vi "CD Init_Prepare Async Data.vi"(8 "error in (no error)":errorcluster, 10 "Card Parameters (in)":T1, 11 "Channels In":T15[](array[typedef]) {"RTs"."Mode Codes"."Words Item Refs" format="%.0x"; "RTs"."Mode Codes"."Timestamp Channel Data Reference" format="%.0x"; "RTs"."subAddresses"."Words Item Refs" format="%.0x"; "RTs"."subAddresses"."Timestamp Channel Data Reference" format="%.0x"; "RTs"."Status Channel Data Reference" format="%.0x"; "RTs"."Command Channels Refs" format="%.0x"; "BC"."Acyclic Frames Trigger Channels Refs" format="%.0x"; "BC"."Command Channels Refs" format="%.0x"; "BC"."messages"."Timestamp Channel Data Reference" format="%.0x"; "BC"."messages"."Status Channel Data Refs" format="%.0x"; "BC"."messages"."Words Item Refs" format="%.0x"; "BC"."messages"."Words Block Data Refs"."Data Reference" format="%.0x"}) -> (0 "error out":errorcluster, 3 "RT Async Data":T3 {"Map (MC Tx)"."Word Data Reference" format="%.0x"; "Map (MC Rx)"."Channel Data Reference" format="%.0x"; "Map (RT Command Channels)"."RT Command Channel Ref" format="%.0x"; "MAP (BC Acyclic Messages Trigger)"."Acyclic Message Trigger Channel Ref" format="%.0x"; "Map (Bc Command Channels)"."BC Command Channel Ref" format="%.0x"; "Map (RT to ..)"."Word Data Reference" format="%.0x"; "Map (BC to RT)"."Channel Data Reference" format="%.0x"})   [LabVIEW 2017, in "Ballard MIL-1553 Engine.lvlib"]
uses:
  Ballard MIL-1553 Engine.lvlib
  Shared/Controls and Global/RT Channel.ctl
  Shared/Controls and Global/RT BC.ctl
  <vilib>/NI Veristand/Custom Device API/Custom Device Item Ref.ctl
  Shared/Controls and Global/RT Message.ctl
  Shared/Controls and Global/RT messageType.ctl
  Shared/Controls and Global/RT CWD1.ctl
  Shared/Controls and Global/RT CWD2.ctl
  <vilib>/NI Veristand/Custom Device API/Data Reference.ctl
  <vilib>/NI Veristand/Custom Device API/Block Data Reference.ctl
  Shared/Controls and Global/RT Remote Terminal.ctl
  Shared/Controls and Global/RT Remote Terminal_rtMode.ctl
  Shared/Controls and Global/RT Remote Terminal_RT subAddress.ctl
  Shared/Controls and Global/RT Remote Terminal_RT direction.ctl
  Shared/Controls and Global/RT Remote Terminal_RT Mode Code.ctl
  Controls/RT Async Data.ctl
  Controls/RT Async_Map BC2RT.ctl
  Controls/RT Async_Map_Type.ctl
  Controls/RT Async_Raw Values.ctl
  Controls/RT Async_Raw Values to Messages Index_Association.ctl
  Controls/RT Async_Map RT2BC.ctl
  Controls/RT Async_Map RTs Status.ctl
  Controls/RT Async_Map BC Command Channels.ctl
  Controls/RT Async_Map BC Acyclic Messages Trigger.ctl
  Controls/RT Async_Map RT Command Channels.ctl
  Controls/Card Parameters.ctl
  Shared/Controls and Global/Initialization Method.ctl
  <vilib>/NI VeriStand/Custom Device API/Custom Device API.lvlib
  Shared/Ballard 1553 Shared.lvlib
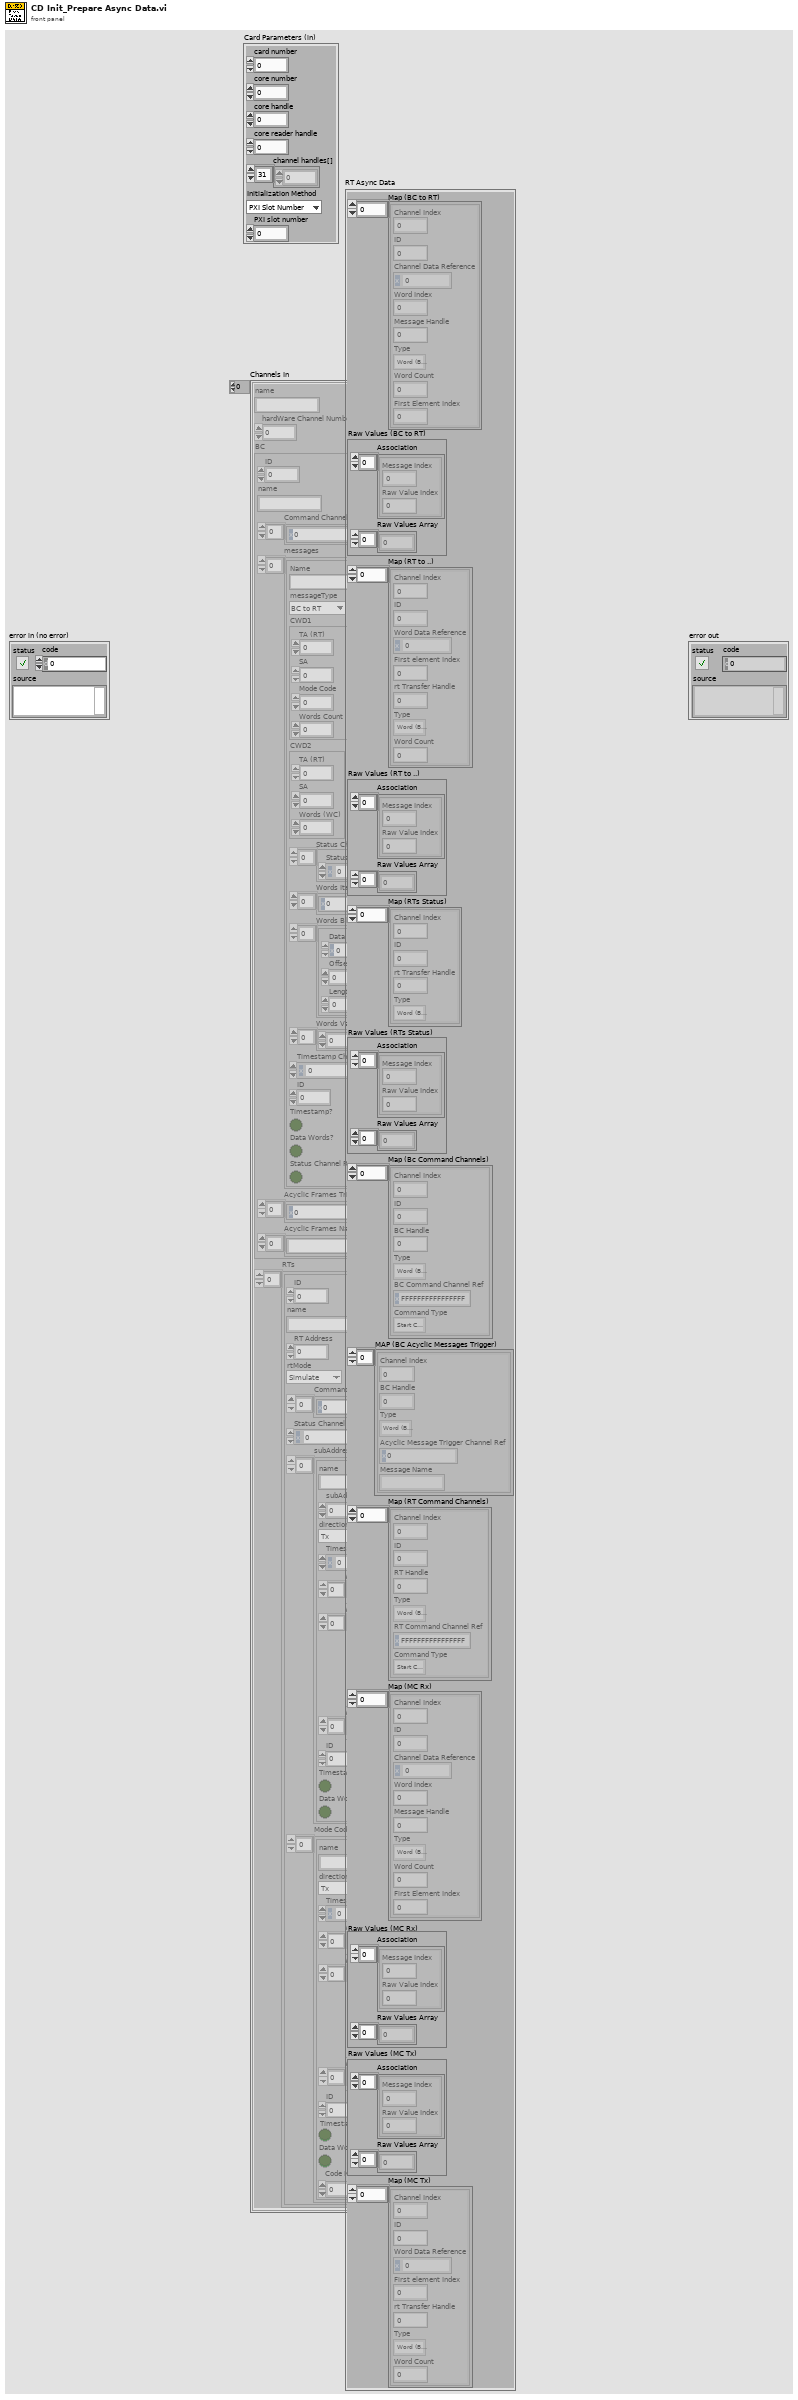
[diagram p1: front panel]
types:
  T1 = typedef "Ballard MIL-1553 Engine.lvlib/Card Parameters.ctl" = cluster{"card number":i32, "core number":i32, "core handle":u64, "core reader handle":u64, "channel handles[]":u64[], "Initialization Method":T2, "PXI slot number":i32}
  T2 = typedef "Ballard 1553 Shared.lvlib/Initialization Method.ctl" = enum16{"PXI Slot Number", "Card Number"}
  T3 = typedef "Ballard MIL-1553 Engine.lvlib/RT Async Data.ctl" = cluster{"Map (BC to RT)":T4[], "Raw Values (BC to RT)":T7, "Map (RT to ..)":T9[], "Raw Values (RT to ..)":T7, "Map (RTs Status)":T10[], "Raw Values (RTs Status)":T7, "Map (Bc Command Channels)":T11[], "MAP (BC Acyclic Messages Trigger)":T13[], "Map (RT Command Channels)":T14[], "Map (MC Rx)":T4[], "Raw Values (MC Rx)":T7, "Raw Values (MC Tx)":T7, "Map (MC Tx)":T9[]}
  T4 = typedef "Ballard MIL-1553 Engine.lvlib/RT Async_Map BC2RT.ctl" = cluster{"Channel Index":i32, "ID":i32, "Channel Data Reference":T5, "Word Index":i32, "Message Handle":u64, "Type":T6, "Word Count":i32, "First Element Index":i32}
  T5 = typedef "Custom Device API.lvlib/Data Reference.ctl" = i32
  T6 = typedef "Ballard MIL-1553 Engine.lvlib/RT Async_Map_Type.ctl" = enum16{"Word (BC to RT)", "Word (MC (Rx))", "Acyclic Message Trigger", "Word (RT to ..)", "Word (RT to RT)", "Word (MC (Tx))", "RT Status", "BC Commands", "RT Commands"}
  T7 = typedef "Ballard MIL-1553 Engine.lvlib/RT Async_Raw Values.ctl" = cluster{"Association":T8[], "Raw Values Array":u16[]}
  T8 = typedef "Ballard MIL-1553 Engine.lvlib/RT Async_Raw Values to Messages Index_Association.ctl" = cluster{"Message Index":i32, "Raw Value Index":i32}
  T9 = typedef "Ballard MIL-1553 Engine.lvlib/RT Async_Map RT2BC.ctl" = cluster{"Channel Index":i32, "ID":i32, "Word Data Reference":T5, "First element Index":i32, "rt Transfer Handle":u64, "Type":T6, "Word Count":i32}
  T10 = typedef "Ballard MIL-1553 Engine.lvlib/RT Async_Map RTs Status.ctl" = cluster{"Channel Index":i32, "ID":i32, "rt Transfer Handle":u64, "Type":T6}
  T11 = typedef "Ballard MIL-1553 Engine.lvlib/RT Async_Map BC Command Channels.ctl" = cluster{"Channel Index":i32, "ID":i32, "BC Handle":u64, "Type":T6, "BC Command Channel Ref":T12, "Command Type":enum16{"Start Command", "Stop Command"}}
  T12 = typedef "Custom Device API.lvlib/Custom Device Item Ref.ctl" = u64
  T13 = typedef "Ballard MIL-1553 Engine.lvlib/RT Async_Map BC Acyclic Messages Trigger.ctl" = cluster{"Channel Index":i32, "BC Handle":u64, "Type":T6, "Acyclic Message Trigger Channel Ref":T12, "Message Name":string}
  T14 = typedef "Ballard MIL-1553 Engine.lvlib/RT Async_Map RT Command Channels.ctl" = cluster{"Channel Index":i32, "ID":i32, "RT Handle":u64, "Type":T6, "RT Command Channel Ref":T12, "Command Type":enum16{"Start Command", "Stop Command"}}
  T15 = typedef "Ballard 1553 Shared.lvlib/RT Channel.ctl" = cluster{"name":string, "hardWare Channel Number":u16, "BC":T16, "RTs":T22[]}
  T16 = typedef "Ballard 1553 Shared.lvlib/RT BC.ctl" = cluster{"ID":i32, "name":string, "Command Channels Refs":T12[], "messages":T17[], "Acyclic Frames Trigger Channels Refs":T12[], "Acyclic Frames Names":string[]}
  T17 = typedef "Ballard 1553 Shared.lvlib/RT Message.ctl" = cluster{"Name":string, "messageType":T18, "CWD1":T19, "CWD2":T20, "Status Channel Data Refs":T5[], "Words Item Refs":T12[], "Words Block Data Refs":T21[], "Words Values Array":u16[], "Timestamp Channel Data Reference":T5, "ID":i32, "Timestamp?":bool, "Data Words?":bool, "Status Channel Ref?":bool}
  T18 = typedef "Ballard 1553 Shared.lvlib/RT messageType.ctl" = enum16{"BC to RT", "RT to BC", "RT to RT", "MC (Rx)", "MC (Tx)"}
  T19 = typedef "Ballard 1553 Shared.lvlib/RT CWD1.ctl" = cluster{"TA (RT)":i8, "SA":i8, "Mode Code":i8, "Words Count":i8}
  T20 = typedef "Ballard 1553 Shared.lvlib/RT CWD2.ctl" = cluster{"TA (RT)":i8, "SA":i8, "Words (WC)":i8}
  T21 = typedef "Custom Device API.lvlib/Block Data Reference.ctl" = cluster{"Data Reference":T5, "Offset":u64, "Length":u64}
  T22 = typedef "Ballard 1553 Shared.lvlib/RT Remote Terminal.ctl" = cluster{"ID":i32, "name":string, "RT Address":i32, "rtMode":T23, "Command Channels Refs":T12[], "Status Channel Data Reference":T5, "subAddresses":T24[], "Mode Codes":T26[]}
  T23 = typedef "Ballard 1553 Shared.lvlib/RT Remote Terminal_rtMode.ctl" = enum16{"Simulate", "Monitor", "Disable"}
  T24 = typedef "Ballard 1553 Shared.lvlib/RT Remote Terminal_RT subAddress.ctl" = cluster{"name":string, "subAddress":i8, "direction":T25, "Timestamp Channel Data Reference":T5, "Words Values Array":u16[], "Words Block Data Refs":T21[], "Words Item Refs":T12[], "ID":i32, "Timestamp?":bool, "Data Words?":bool}
  T25 = typedef "Ballard 1553 Shared.lvlib/RT Remote Terminal_RT direction.ctl" = enum16{"Tx", "Rx"}
  T26 = typedef "Ballard 1553 Shared.lvlib/RT Remote Terminal_RT Mode Code.ctl" = cluster{"name":string, "direction":T25, "Timestamp Channel Data Reference":T5, "Words Values Array":u16[], "Words Block Data Refs":T21[], "Words Item Refs":T12[], "ID":i32, "Timestamp?":bool, "Data Words?":bool, "Code Number":i32}
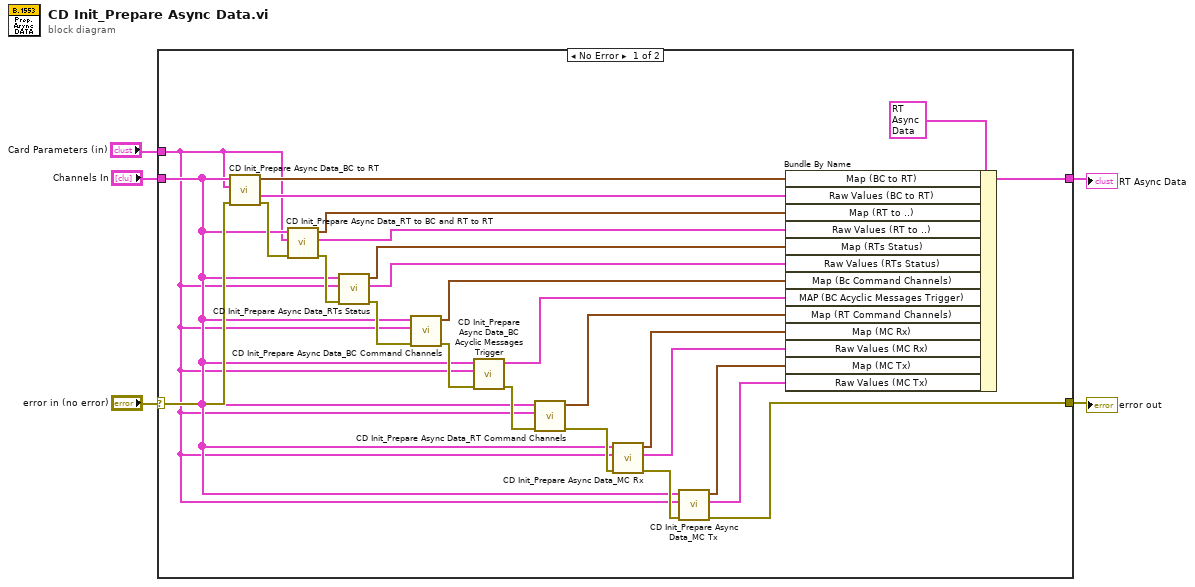
[diagram p0: block diagram]
diagram:
  n1 = case shown="No Error" "error in (no error)" {
    selector: "error in (no error)" -> [w30 w32]
    tunnel: [w10 w32] -> w4
    tunnel: "Channels In" -> [w7 _]
    tunnel: "Card Parameters (in)" -> [w6 _]
    tunnel: [w31 _] -> w1
    frame No Error {
      n2 = call "CD Init_Prepare Async Data_BC to RT.vi"("error in (no error)"=w30, "Card Parameters (in)"=w6, "Channels In"=w7) -> ("error out"=w24:errorcluster, "Raw Values (BC to RT)"=w27:T7, "Map (BC to RT)"=w28:T4[])  [unwired: 6 in]
      n3 = call "CD Init_Prepare Async Data_RT to BC and RT to RT.vi"("error in (no error)"=w24, "Card Parameters (in)"=w6, "Channels In"=w7) -> ("error out"=w23:errorcluster, "Raw Values (RT to BC)"=w25:T7, "Map (RT to BC)"=w26:T9[])  [unwired: 6 in]
      n4 = call "CD Init_Prepare Async Data_RTs Status.vi"("error in (no error)"=w23, "Card Parameters (in)"=w6, "Channels In"=w7) -> ("error out"=w20:errorcluster, "Raw Values (RTs Status)"=w21:T7, "Map (RTs Status)"=w22:T10[])  [unwired: 6 in]
      n5 = call "CD Init_Prepare Async Data_BC Command Channels.vi"("error in (no error)"=w20, "Card Parameters (in)"=w6, "Channels In"=w7) -> ("error out"=w18:errorcluster, "Map (Bc Command Channels)"=w19:T11[])  [unwired: 7 in]
      n6 = call "CD Init_Prepare Async Data_BC Acyclic Messages Trigger.vi"("error in (no error)"=w18, "Card Parameters (in)"=w6, "Channels In"=w7) -> ("error out"=w17:errorcluster, "MAP (BC Acyclic Messages Trigger)"=w16:T13[])  [unwired: 7 in]
      n7 = call "CD Init_Prepare Async Data_RT Command Channels.vi"("error in (no error)"=w17, "Card Parameters (in)"=w6, "Channels In"=w7) -> ("error out"=w14:errorcluster, "Map (RT Command Channels)"=w15:T14[])  [unwired: 7 in]
      n8 = call "CD Init_Prepare Async Data_MC Rx.vi"("error in (no error)"=w14, "Card Parameters (in)"=w6, "Channels In"=w7) -> ("error out"=w11:errorcluster, "Raw Values (MC Rx)"=w12:T7, "Map (MC Rx)"=w13:T4[])  [unwired: 6 in]
      n9 = call "CD Init_Prepare Async Data_MC Tx.vi"("error in (no error)"=w11, "Card Parameters (in)"=w6, "Channels In"=w7) -> ("error out"=w10:errorcluster, "Raw Values (RT to BC)"=w8:T7, "Map (MC Tx)"=w9:T9[])  [unwired: 6 in]
      n10 = Bundle By Name(cluster=T3 {"Map (BC to RT)"=[], "Raw Values (BC to RT)"={"Association"=[], "Raw Values Array"=[]}, "Map (RT to ..)"=[], "Raw Values (RT to ..)"={"Association"=[], "Raw Values Array"=[]}, "Map (RTs Status)"=[], "Raw Values (RTs Status)"={"Association"=[], "Raw Values Array"=[]}, "Map (Bc Command Channels)"=[], "MAP (BC Acyclic Messages Trigger)"=[], "Map (RT Command Channels)"=[], "Map (MC Rx)"=[], "Raw Values (MC Rx)"={"Association"=[], "Raw Values Array"=[]}, "Raw Values (MC Tx)"={"Association"=[], "Raw Values Array"=[]}, "Map (MC Tx)"=[]} ("RT Async Data"), "Map (BC to RT)"=w28, "Raw Values (BC to RT)"=w27, "Map (RT to ..)"=w26, "Raw Values (RT to ..)"=w25, "Map (RTs Status)"=w22, "Raw Values (RTs Status)"=w21, "Map (Bc Command Channels)"=w19, "MAP (BC Acyclic Messages Trigger)"=w16, "Map (RT Command Channels)"=w15, "Map (MC Rx)"=w13, "Raw Values (MC Rx)"=w12, "Map (MC Tx)"=w9, "Raw Values (MC Tx)"=w8) -> (w31:T3)
    }
    frame Error {
    }
  }
  "error out" <- w4
  "RT Async Data" <- w1
